vi "Get Event Timeout.vi"(11 "HL Timer in":refnum<class "Loop Timer.lvclass">) -> (2 "Event Timeout":i32, 3 "HL Timer out":refnum<class "Loop Timer.lvclass">)   [LabVIEW 2022 SP3, in "hse-misc.lvlib" / "Loop Timer.lvclass"]
doc: "____\nHAMPEL SOFTWARE ENGINEERING v3.8.0 (2023-12-18 14:41)"
uses:
  Loop Timer.lvclass
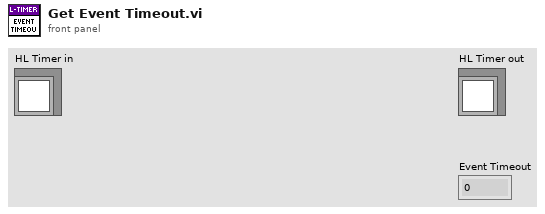
[diagram p1: front panel]
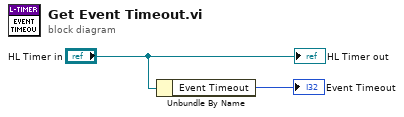
[diagram p0: block diagram]
diagram:
  n1 = Unbundle By Name("HL Timer in") -> ("Event Timeout"=→"Event Timeout":i32)
  "HL Timer out" <- "HL Timer in"
